vi "Day 16.vi"() -> ()   [LabVIEW 2023]
uses:
  <vilib>/Utility/error.llb/Trim Whitespace One-Sided.vi
panel:
  in  "time left":i32=30
  out "most pressure":i32
  in  "test":bool
  in  "test input":string="Valve AA has flow rate=0; tunnels lead to valves DD, II, BB\nValve BB has flow rate=13; tunnels lead to valves CC, AA\nValve CC has flow rate=2; tunnels lead to valves DD, BB\nValve DD has flow rate=20; tunnels lead to valves CC, AA, EE\nValve EE has flow rate=3; tunnels lead to valves FF, DD\nValve FF has flow rate=0; tunnels lead to valves EE, GG\nValve GG has flow rate=0; tunnels lead to valves FF, HH\nValve HH has flow rate=22; tunnel leads to valve GG\nValve II has flow rate=0; tunnels lead to valves AA, JJ\nValve JJ has flow rate=21; tunnel leads to valve II"
  in  "input":string="Valve DR has flow rate=22; tunnels lead to valves DC, YA\nValve IO has flow rate=14; tunnels lead to valves GE, CK, HY, XB\nValve XY has flow rate=0; tunnels lead to valves IP, AR\nValve UQ has flow rate=0; tunnels lead to valves XU, PD\nValve FO has flow rate=0; tunnels lead to valves DL, NC\nValve PU has flow rate=0; tunnels lead to valves ZJ, AN\nValve MK has flow rate=0; tunnels lead to valves ZS, SB\nValve HN has flow rate=0; tunnels lead to valves AA, DV\nValve XF has flow rate=0; tunnels lead to valves XB, AA\nValve OD has flow rate=13; tunnels lead to valves ZS, AF, SY, QQ, AR\nValve GE has flow rate=0; tunnels lead to valves KR, IO\nValve UF has flow rate=18; tunnels lead to valves QQ, AN, YE, GY\nValve WK has flow rate=19; tunnel leads to valve PQ\nValve PQ has flow rate=0; tunnels lead to valves WK, CW\nValve XU has flow rate=0; tunnels lead to valves DV, UQ\nValve SH has flow rate=0; tunnels lead to valves IP, AA\nValve SY has flow rate=0; tunnels lead to valves ZJ, OD\nValve OU has flow rate=0; tunnels lead to valves CK, DL\nValve IP has flow rate=8; tunnels lead to valves CY, ML, YI, XY, SH\nValve XZ has flow rate=0; tunnels lead to valves AM, PD\nValve ZU has flow rate=0; tunnels lead to valves CW, SB\nValve DC has flow rate=0; tunnels lead to valves CF, DR\nValve QY has flow rate=0; tunnels lead to valves CW, MQ\nValve XB has flow rate=0; tunnels lead to valves IO, XF\nValve AF has flow rate=0; tunnels lead to valves PD, OD\nValve GY has flow rate=0; tunnels lead to valves UF, ZC\nValve ZC has flow rate=0; tunnels lead to valves GY, CW\nValve ZJ has flow rate=25; tunnels lead to valves SY, PU\nValve NC has flow rate=6; tunnels lead to valves HY, ML, NJ, AT, FO\nValve DS has flow rate=0; tunnels lead to valves AT, DV\nValve DV has flow rate=7; tunnels lead to valves FD, KR, HN, DS, XU\nValve HY has flow rate=0; tunnels lead to valves NC, IO\nValve WF has flow rate=0; tunnels lead to valves NJ, AA\nValve CK has flow rate=0; tunnels lead to valves IO, OU\nValve YE has flow rate=0; tunnels lead to valves CY, UF\nValve LA has flow rate=0; tunnels lead to valves DL, ZM\nValve QQ has flow rate=0; tunnels lead to valves OD, UF\nValve AM has flow rate=0; tunnels lead to valves XZ, SB\nValve AN has flow rate=0; tunnels lead to valves UF, PU\nValve CL has flow rate=16; tunnels lead to valves YA, LD\nValve CF has flow rate=12; tunnel leads to valve DC\nValve FD has flow rate=0; tunnels lead to valves DV, DL\nValve QU has flow rate=0; tunnels lead to valves LD, PD\nValve AT has flow rate=0; tunnels lead to valves DS, NC\nValve SB has flow rate=24; tunnels lead to valves MK, AM, ZU\nValve YI has flow rate=0; tunnels lead to valves DL, IP\nValve ZM has flow rate=0; tunnels lead to valves AA, LA\nValve LD has flow rate=0; tunnels lead to valves CL, QU\nValve AR has flow rate=0; tunnels lead to valves OD, XY\nValve DL has flow rate=5; tunnels lead to valves FO, LA, YI, OU, FD\nValve MQ has flow rate=0; tunnels lead to valves QY, PD\nValve PD has flow rate=9; tunnels lead to valves MQ, QU, XZ, AF, UQ\nValve KR has flow rate=0; tunnels lead to valves GE, DV\nValve CY has flow rate=0; tunnels lead to valves YE, IP\nValve AA has flow rate=0; tunnels lead to valves SH, XF, ZM, HN, WF\nValve NJ has flow rate=0; tunnels lead to valves NC, WF\nValve YA has flow rate=0; tunnels lead to valves CL, DR\nValve ML has flow rate=0; tunnels lead to valves NC, IP\nValve CW has flow rate=15; tunnels lead to valves QY, PQ, ZC, ZU\nValve ZS has flow rate=0; tunnels lead to valves MK, OD\n"
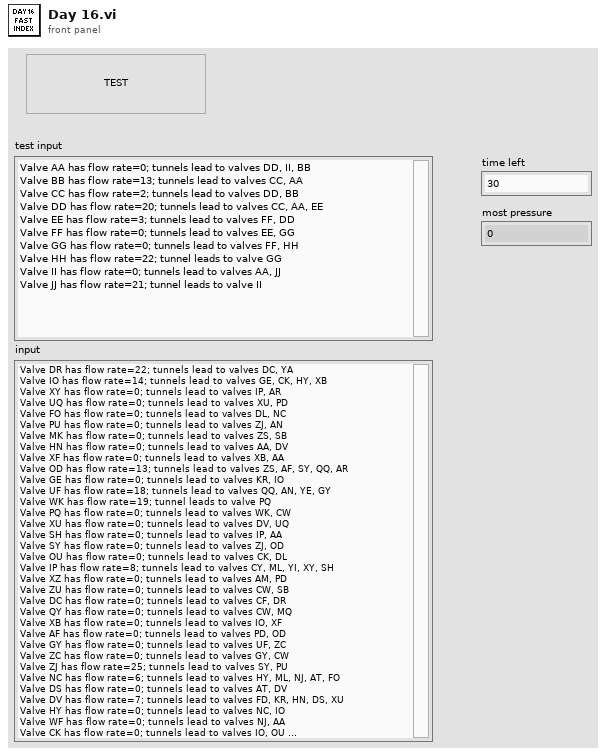
[diagram p1: front panel]
types:
  T1 = cluster{"bitfield":u32, "time left":i32, "index":i32}
  T2 = cluster{"distance[]":cluster{"index":i32, "distance":i32}[], "index":i32}
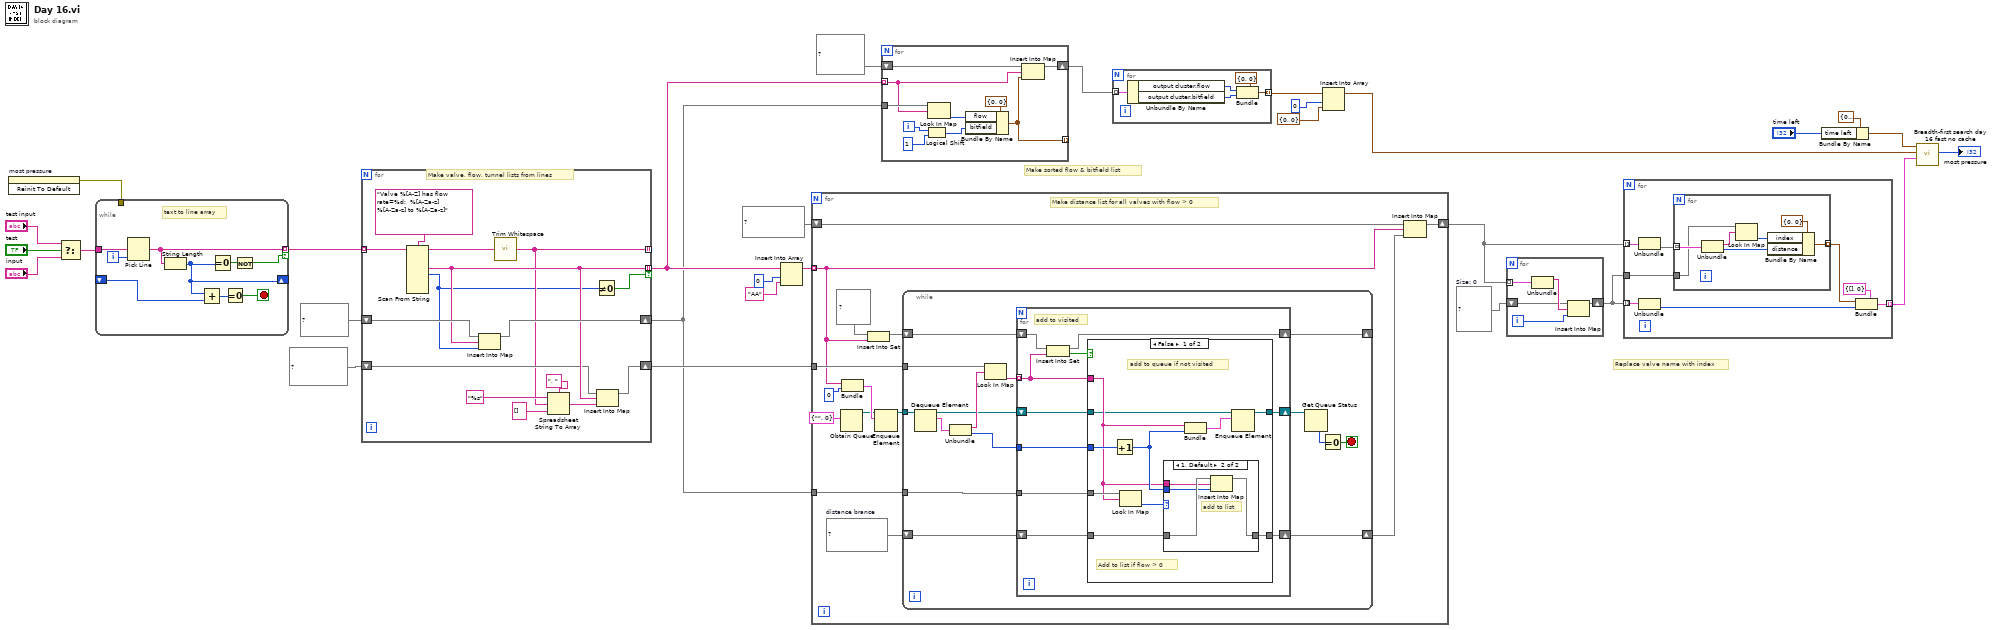
[diagram p0: block diagram]
diagram:
  w12 = map{string, i32} {}  # Size: 0
  # "Replace valve name with index"
  # "Make sorted flow & bitfield list"
  n1 = invoke on="most pressure" class="DigNum (strict)" method="Reinit To Default"() -> (error out=w1:errorcluster)  [unwired: 3 in, 2 out]
  n2 = Select(t="test input", s="test", f="input") -> (s? t:f=w26:string)
  n3 = while {
    tunnel: w26 -> [w37]
    tunnel: [w30] -> w27 mode=indexing if=w36
    shift-right: [w33] -> _
    shift-left: _ -> [w34]
    tunnel: w1 -> [_]
    i -> [w38]
    stop <- w31 stop-if-true
    # "text to line array"
    n4 = Pick Line(multi-line string=w37, line index=w38) -> (output string=w30:string)  [unwired: 1 in]
    n5 = String Length(string=w30) -> (length=w33:i32)
    n6 = Add(x=w33, y=w34) -> (x+y=w35:i32)
    n7 = Equal To 0?(x=w33) -> (x = 0?=w32:bool)
    n8 = Equal To 0?(x=w35) -> (x = 0?=w31:bool)
    n9 = Not(x=w32) -> (.not. x?=w36:bool)
  }
  n10 = for {
    tunnel: w27 -> [w53] mode=indexing
    tunnel: [w49] -> w16 mode=indexing if=w40
    tunnel: [w41] -> _ mode=indexing
    shift-right: [w51] -> w15
    shift-left: map{string, i32} {} ("Size: 0") -> [w50]
    shift-right: [w44] -> w19
    shift-left: map{string, string[]} {} ("Size: 0") -> [w43]
    # "Make valve, flow, tunnel lists from lines"
    n11 = Scan From String(format string="Valve %[A-Z] has flow rate=%d;  %[A-Za-z] %[A-Za-z] to %[A-Za-z]", input string=w53) -> (remaining string=w46:string, output 1=w49:string, output 2=w39:i32)  [unwired: 10 in, 2 out]
    n12 = Insert Into Map(map in=w50, key=w49, value=w39) -> (map out=w51:map{string, i32})  [unwired: 2 out]
    n13 = call <vilib>:"Trim Whitespace.vi"("string"=w46) -> ("trimmed string"=w41:string)  [unwired: 1 in]
    n14 = Spreadsheet String To Array(delimiter (Tab)=", ", format string="%s", spreadsheet string=w41, array type (2D Dbl)=string[] [] ("appended array")) -> (array=w48:string[])
    n15 = Not Equal To 0?(x=w39) -> (x != 0?=w40:bool)
    n16 = Insert Into Map(map in=w43, key=w49, value=w48) -> (map out=w44:map{string, string[]})  [unwired: 2 out]
  }
  n17 = Insert Into Array(array=w16, index=0, new element="AA" ("new element/subarray")) -> (w20:string[])
  n18 = for {
    tunnel: w19 -> [w65]
    tunnel: w15 -> [w66]
    tunnel: w20 -> [w60] mode=indexing
    shift-right: [w62] -> w13
    shift-left: map{string, map{string, i32}} {} ("Size: 0") -> [w63]
    w56 = map{string, i32} {}  # distance brance
    # "Make distance list for all valves with flow > 0"
    n19 = Obtain Queue(element data type=cluster{string, i32} {"", 0} ("output cluster")) -> (queue out=w54:refnum<queue>)  [unwired: 4 in, 2 out]
    n20 = Bundle(w60, "x+1"=0) -> (w58:cluster{string, "x+1":i32})  [unwired: 1 in]
    n21 = Insert Into Set(10:w60, 11:set{string} {} ("Size: 0")) -> (3:w67:set{string})  [unwired: 1 out]
    n22 = Enqueue Element(queue=w54, element=w58) -> (queue out=w61:refnum<queue>)  [unwired: 2 in, 2 out]
    n23 = while {
      tunnel: w66 -> [w80]
      shift-right: [w81] -> _
      shift-left: w67 -> [w82]
      shift-right: [w79] -> w64
      shift-left: w56 -> [w78]
      tunnel: w65 -> [w77]
      tunnel: w61 -> [w75]
      stop <- w69 stop-if-true
      n24 = Dequeue Element(queue=w75) -> (queue out=w71:refnum<queue>, element=w74:cluster{string, i32})  [unwired: 2 in, 2 out]
      n25 = Unbundle(w74) -> (w73:string, w72:i32)
      n26 = Look In Map(map=w77, key=w73) -> (value=w76:string[])  [unwired: 1 in, 1 out]
      n27 = for {
        tunnel: w76 -> [w87] mode=indexing
        shift-right: [w91] -> w81
        shift-left: w82 -> [w92]
        tunnel: w80 -> [w89]
        tunnel: w72 -> [w88]
        shift-right: [w86] -> w79
        shift-left: w78 -> [w85]
        shift-right: [w83] -> w70
        shift-left: w71 -> [w84]
        # "add to visited"
        n28 = Insert Into Set(10:w87, 11:w92) -> (2:w90:bool, 3:w91:set{string})
        n29 = case shown="False" w90 {
          tunnel: w89 -> [w102 _]
          tunnel: w88 -> [w98 _]
          tunnel: w87 -> [w96 _]
          tunnel: [w100 w109] -> w86
          tunnel: w85 -> [w99 w109]
          tunnel: w84 -> [w95 w108]
          tunnel: [w93 w108] -> w83
          frame False {
            # "Add to list if flow > 0"
            # "add to queue if not visited"
            n30 = Increment(x=w98) -> (x+1=w97:i32)
            n31 = Look In Map(map=w102, key=w96) -> (value=w101:i32)  [unwired: 1 in, 1 out]
            n32 = case shown="1, Default" w101 {
              tunnel: w96 -> [_ w104]
              tunnel: [w103 w106] -> w100
              tunnel: w99 -> [w103 w107]
              tunnel: w97 -> [_ w105]
              frame 0 {
              }
              frame 1, Default {
                # "add to list"
                n33 = Insert Into Map(map in=w107, key=w104, value=w105) -> (map out=w106:map{string, i32})  [unwired: 2 out]
              }
            }
            n34 = Bundle(w96, w97) -> (w94:cluster{string, i32})  [unwired: 1 in]
            n35 = Enqueue Element(queue=w95, element=w94) -> (queue out=w93:refnum<queue>)  [unwired: 2 in, 2 out]
          }
          frame True {
          }
        }
      }
      n36 = Get Queue Status(queue=w70) -> (# elements in queue=w68:i32)  [unwired: 2 in, 7 out]
      n37 = Equal To 0?(x=w68) -> (x = 0?=w69:bool)
    }
    n38 = Insert Into Map(map in=w63, key=w60, value=w64) -> (map out=w62:map{string, map{string, i32}})  [unwired: 2 out]
  }
  n39 = for {
    tunnel: w16 -> [w111] mode=indexing
    tunnel: w15 -> [w115]
    shift-right: [w113] -> w4
    shift-left: map{string, cluster{"flow":i32, "bitfield":u32}} {} ("Size: 0") -> [w112]
    tunnel: [w110] -> _ mode=indexing
    i -> [w118]
    n40 = Logical Shift(y=w118, x=u32 1) -> (x << y=w116:u32)
    n41 = Look In Map(map=w115, key=w111) -> (value=w117:i32)  [unwired: 1 in, 1 out]
    n42 = Bundle By Name(cluster=cluster{"flow":i32, "bitfield":u32} {"flow"=0, "bitfield"=0} ("output cluster"), "flow"=w117, "bitfield"=w116) -> (w110:cluster{"flow":i32, "bitfield":u32})
    n43 = Insert Into Map(map in=w112, key=w111, value=w110) -> (map out=w113:map{string, cluster{"flow":i32, "bitfield":u32}})  [unwired: 2 out]
  }
  n44 = for {
    tunnel: w4 -> [w124] mode=indexing
    tunnel: [w121] -> w6 mode=indexing
    n45 = Unbundle By Name(w124) -> ("output cluster.flow"=w123:i32, "output cluster.bitfield"=w122:u32)
    n46 = Bundle(cluster=cluster{"flow":i32, "bitfield":u32} {"flow"=0, "bitfield"=0}, "flow"=w123, "bitfield"=w122) -> (w121:cluster{"flow":i32, "bitfield":u32})
  }
  n47 = Insert Into Array(array=w6, index=0, new element=cluster{"flow":i32, "bitfield":u32} {"flow"=0, "bitfield"=0} ("output cluster")) -> (w9:cluster{"flow":i32, "bitfield":u32}[])
  n48 = for {
    tunnel: w13 -> [w129] mode=indexing
    shift-right: [w126] -> w11
    shift-left: w12 -> [w125]
    i -> [w127]
    n49 = Unbundle(w129) -> (w128:string)  [unwired: 1 out]
    n50 = Insert Into Map(map in=w125, key=w128, value=w127) -> (map out=w126:map{string, i32})  [unwired: 2 out]
  }
  n51 = for {
    tunnel: w13 -> [w137] mode=indexing
    tunnel: w11 -> [w135] mode=indexing
    tunnel: [w133] -> w10 mode=indexing
    tunnel: w11 -> [w131]
    n52 = Unbundle(w137) -> (w136:map{string, i32})  [unwired: 1 out]
    n53 = Unbundle(w135) -> (w134:i32)  [unwired: 1 out]
    n54 = for {
      tunnel: w136 -> [w144] mode=indexing
      tunnel: [w141] -> w130 mode=indexing
      tunnel: w131 -> [w139]
      n55 = Unbundle(w144) -> ("valve"=w140:string, "distance"=w143:i32)
      n56 = Look In Map(map=w139, key=w140) -> (value=w138:i32)  [unwired: 1 in, 1 out]
      n57 = Bundle By Name(cluster=cluster{"index":i32, "distance":i32} {"index"=0, "distance"=0} ("output cluster"), "index"=w138, "distance"=w143) -> (w141:cluster{"index":i32, "distance":i32})
    }
    n58 = Bundle(cluster=T2 {"distance[]"=[], "index"=0} ("output cluster"), "distance[]"=w130, "index"=w134) -> (w133:T2)
  }
  n59 = Bundle By Name(cluster=T1 {"bitfield"=0, "time left"=0, "index"=0} ("input \n[index, bitfield, time left]"), "time left"="time left") -> (w3:T1)
  n60 = call "Breadth-first search day 16 fast no cache.vi"("distance graph"=w10, "Flow, bitfield"=w9, "input \n[index, bitfield, time left]"=w3) -> ("most pressure"=→"most pressure":i32)  [unwired: 8 in]
